vi "measure_test.vi"() -> ()   [LabVIEW 2019]
panel:
  in  "dir & target 13":T1 {"Target (cm||deg)" format="%#_13g"}
  in  "dir & target 12":T1 {"Target (cm||deg)" format="%#_13g"}
  in  "dir & target 11":T1 {"Target (cm||deg)" format="%#_13g"}
  in  "dir & target 10":T1 {"Target (cm||deg)" format="%#_13g"}
  in  "dir & target 9":T1 {"Target (cm||deg)" format="%#_13g"}
  in  "dir & target 8":T1 {"Target (cm||deg)" format="%#_13g"}
  in  "dir & target 7":T1={"direction"=enum."Tilt(R)", "Target (cm||deg)"=-73.0} {"Target (cm||deg)" format="%#_13g"}
  in  "dir & target 6":T1={"direction"=enum."Tilt(R)", "Target (cm||deg)"=-73.0} {"Target (cm||deg)" format="%#_13g"}
  in  "dir & target 5":T1={"direction"=enum."Forward", "Target (cm||deg)"=-69.2} {"Target (cm||deg)" format="%#_13g"}
  in  "dir & target 4":T1={"direction"=enum."Tilt(R)", "Target (cm||deg)"=-73.0} {"Target (cm||deg)" format="%#_13g"}
  in  "dir & target 3":T1={"direction"=enum."Forward", "Target (cm||deg)"=-69.2} {"Target (cm||deg)" format="%#_13g"}
  in  "dir & target 2":T1={"direction"=enum."Tilt(R)", "Target (cm||deg)"=122.0} {"Target (cm||deg)" format="%#_13g"}
  in  "dir & target 1":T1={"direction"=enum."Tilt(R)", "Target (cm||deg)"=-128.0} {"Target (cm||deg)" format="%#_13g"}
  in  "dir & target":T1={"direction"=enum."Forward", "Target (cm||deg)"=307.0} {"Target (cm||deg)" format="%#_13g"}
  out "error out":errorcluster
  in  "error in (no error)":errorcluster
  # "Out bridge"
  # "In bridge"
  # "In bridge"
  # "Out bridge"
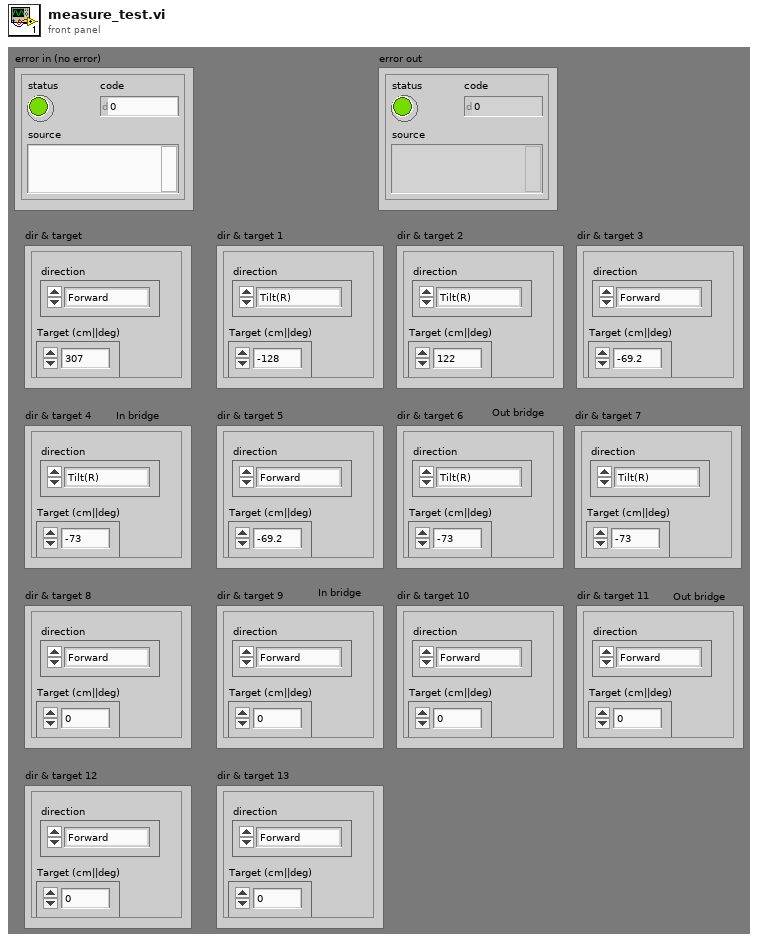
[diagram p1: front panel]
types:
  T1 = cluster{"direction":enum16{"Forward", "Tilt(R)", "Turn"}, "Target (cm||deg)":dbl}
  T2 = enum16{"LeftDown", "LeftUp", "RightDown", "RightUp", "Right", "Left", "Up", "Down", "Middle(X)", "Middle(Y)"}
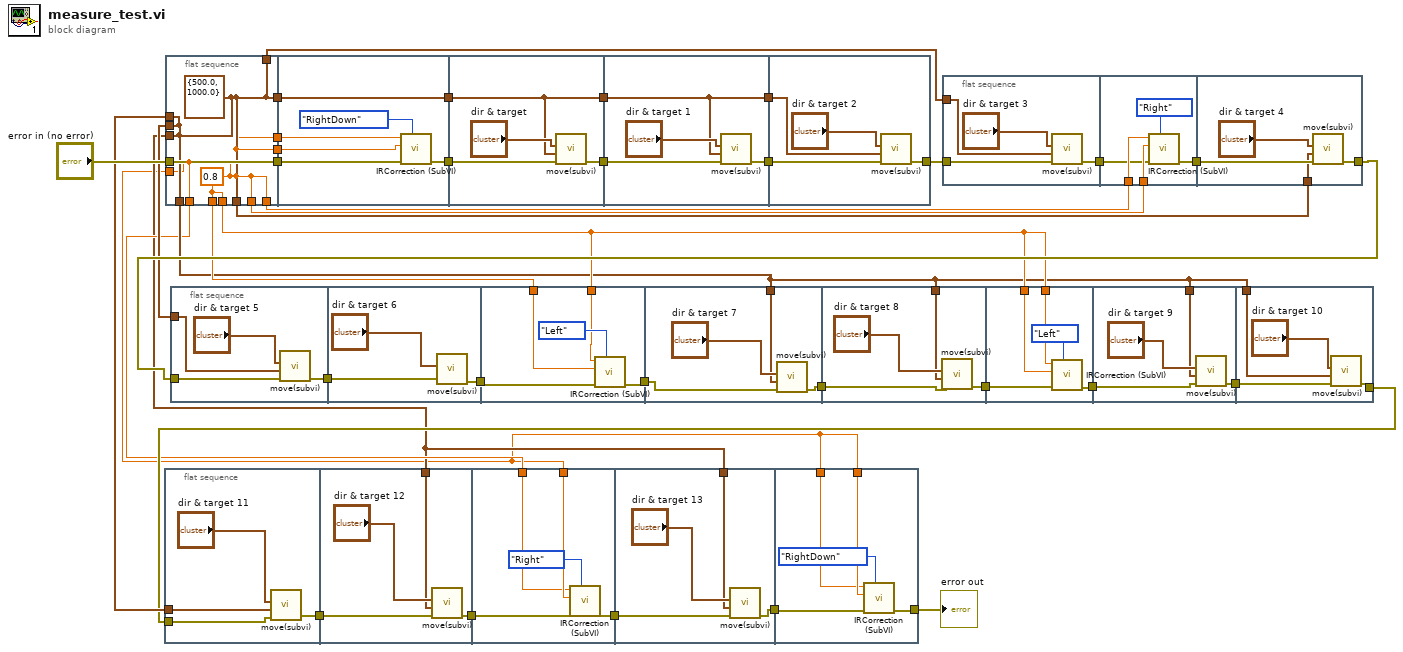
[diagram p0: block diagram]
diagram:
  n1 = flat-sequence {
    tunnel: w10 -> [w43]
    tunnel: w9 -> [w42]
    tunnel: [w41] -> w8
    tunnel: w8 -> [w48]
    tunnel: w3 -> [w46]
    tunnel: [w45] -> w7
    tunnel: w7 -> [w53]
    tunnel: w1 -> [w52]
    tunnel: w6 -> [w51]
    tunnel: [w49] -> w5
    tunnel: w5 -> [w57]
    tunnel: w3 -> [w54]
    tunnel: [w56] -> w2
    tunnel: [w61] -> w4
    tunnel: w2 -> [w62]
    tunnel: w1 -> [w60]
    tunnel: w1 -> [w59]
    frame #0 {
      n2 = call "move(subvi).vi"("Error In"=w42, "speed"=w43, "dir & target"="dir & target 11") -> ("Error Out"=w41:errorcluster)  [unwired: 8 in]
    }
    frame #1 {
      n3 = call "move(subvi).vi"("Error In"=w48, "speed"=w46, "dir & target"="dir & target 12") -> ("Error Out"=w45:errorcluster)  [unwired: 8 in]
    }
    frame #2 {
      n4 = call "IRCorrection (SubVI).vi"("CorrectCorner"=T2."Right", "error in (no error)"=w53, "Y_distance(V)"=w52, "X_distance(V)"=w51) -> ("error out"=w49:errorcluster)  [unwired: 6 in, 1 out]
    }
    frame #3 {
      n5 = call "move(subvi).vi"("Error In"=w57, "speed"=w54, "dir & target"="dir & target 13") -> ("Error Out"=w56:errorcluster)  [unwired: 8 in]
    }
    frame #4 {
      n6 = call "IRCorrection (SubVI).vi"("CorrectCorner"=T2."RightDown", "error in (no error)"=w62, "Y_distance(V)"=w60, "X_distance(V)"=w59) -> ("error out"=w61:errorcluster)  [unwired: 6 in, 1 out]
    }
  }
  n7 = flat-sequence {
    tunnel: [w63] -> w40
    tunnel: [w63] -> w39
    tunnel: "error in (no error)" -> [w65]
    tunnel: [w65] -> w38
    tunnel: [w64] -> w35
    tunnel: [w64] -> w29
    tunnel: [w63] -> w27
    tunnel: [w63] -> w26
    tunnel: [w64] -> w23
    tunnel: [w64] -> w20
    tunnel: [w63] -> w17
    tunnel: [w63] -> w14
    tunnel: [w64] -> w11
    tunnel: [w64] -> w10
    tunnel: [w64] -> w3
    tunnel: [w63] -> w1
    tunnel: [w63] -> w6
    tunnel: w40 -> [w70]
    tunnel: w39 -> [w69]
    tunnel: w38 -> [w68]
    tunnel: [w67] -> w36
    tunnel: w35 -> [w67]
    tunnel: [w66] -> w34
    tunnel: w36 -> [w72]
    tunnel: w34 -> [w74]
    tunnel: [w73] -> w33
    tunnel: [w72] -> w32
    tunnel: w33 -> [w79]
    tunnel: w32 -> [w76]
    tunnel: [w77] -> w31
    tunnel: [w76] -> w30
    tunnel: w31 -> [w83]
    tunnel: w30 -> [w82]
    tunnel: [w80] -> w28
    frame #0 {
      w64 = cluster{"acc (deg/s^2)":dbl, "Vmax (deg/s)":dbl} {"acc (deg/s^2)"=500.0, "Vmax (deg/s)"=1000.0} ("speed")
      w63 = 0.8 ("X_distance(V)")
    }
    frame #1 {
      n8 = call "IRCorrection (SubVI).vi"("CorrectCorner"=T2."RightDown", "error in (no error)"=w68, "Y_distance(V)"=w69, "X_distance(V)"=w70) -> ("error out"=w66:errorcluster)  [unwired: 6 in, 1 out]
    }
    frame #2 {
      n9 = call "move(subvi).vi"("Error In"=w74, "speed"=w72, "dir & target"="dir & target") -> ("Error Out"=w73:errorcluster)  [unwired: 8 in]
    }
    frame #3 {
      n10 = call "move(subvi).vi"("Error In"=w79, "speed"=w76, "dir & target"="dir & target 1") -> ("Error Out"=w77:errorcluster)  [unwired: 8 in]
    }
    frame #4 {
      n11 = call "move(subvi).vi"("Error In"=w83, "speed"=w82, "dir & target"="dir & target 2") -> ("Error Out"=w80:errorcluster)  [unwired: 8 in]
    }
  }
  n12 = flat-sequence {
    tunnel: w20 -> [w86]
    tunnel: w21 -> [w85]
    tunnel: [w84] -> w22
    tunnel: w22 -> [w89]
    tunnel: [w88] -> w19
    tunnel: w19 -> [w95]
    tunnel: [w94] -> w18
    tunnel: w17 -> [w92]
    tunnel: w14 -> [w91]
    tunnel: w18 -> [w98]
    tunnel: w11 -> [w97]
    tunnel: [w96] -> w16
    tunnel: w16 -> [w103]
    tunnel: w11 -> [w101]
    tunnel: [w100] -> w15
    tunnel: w15 -> [w108]
    tunnel: w14 -> [w107]
    tunnel: w14 -> [w106]
    tunnel: [w105] -> w13
    tunnel: w13 -> [w112]
    tunnel: [w111] -> w12
    tunnel: w11 -> [w109]
    tunnel: w12 -> [w116]
    tunnel: w11 -> [w114]
    tunnel: [w113] -> w9
    frame #0 {
      n13 = call "move(subvi).vi"("Error In"=w85, "speed"=w86, "dir & target"="dir & target 5") -> ("Error Out"=w84:errorcluster)  [unwired: 8 in]
    }
    frame #1 {
      n14 = call "move(subvi).vi"("Error In"=w89, "dir & target"="dir & target 6") -> ("Error Out"=w88:errorcluster)  [unwired: 9 in]
    }
    frame #2 {
      n15 = call "IRCorrection (SubVI).vi"("CorrectCorner"=T2."Left", "error in (no error)"=w95, "Y_distance(V)"=w92, "X_distance(V)"=w91) -> ("error out"=w94:errorcluster)  [unwired: 6 in, 1 out]
    }
    frame #3 {
      n16 = call "move(subvi).vi"("Error In"=w98, "speed"=w97, "dir & target"="dir & target 7") -> ("Error Out"=w96:errorcluster)  [unwired: 8 in]
    }
    frame #4 {
      n17 = call "move(subvi).vi"("Error In"=w103, "speed"=w101, "dir & target"="dir & target 8") -> ("Error Out"=w100:errorcluster)  [unwired: 8 in]
    }
    frame #5 {
      n18 = call "IRCorrection (SubVI).vi"("CorrectCorner"=T2."Left", "error in (no error)"=w108, "Y_distance(V)"=w106, "X_distance(V)"=w107) -> ("error out"=w105:errorcluster)  [unwired: 6 in, 1 out]
    }
    frame #6 {
      n19 = call "move(subvi).vi"("Error In"=w112, "speed"=w109, "dir & target"="dir & target 9") -> ("Error Out"=w111:errorcluster)  [unwired: 8 in]
    }
    frame #7 {
      n20 = call "move(subvi).vi"("Error In"=w116, "speed"=w114, "dir & target"="dir & target 10") -> ("Error Out"=w113:errorcluster)  [unwired: 8 in]
    }
  }
  n21 = flat-sequence {
    tunnel: w29 -> [w119]
    tunnel: w28 -> [w118]
    tunnel: [w117] -> w25
    tunnel: w27 -> [w125]
    tunnel: w26 -> [w124]
    tunnel: w25 -> [w123]
    tunnel: [w122] -> w24
    tunnel: w24 -> [w129]
    tunnel: [w128] -> w21
    tunnel: w23 -> [w126]
    frame #0 {
      n22 = call "move(subvi).vi"("Error In"=w118, "speed"=w119, "dir & target"="dir & target 3") -> ("Error Out"=w117:errorcluster)  [unwired: 8 in]
    }
    frame #1 {
      n23 = call "IRCorrection (SubVI).vi"("CorrectCorner"=T2."Right", "error in (no error)"=w123, "Y_distance(V)"=w124, "X_distance(V)"=w125) -> ("error out"=w122:errorcluster)  [unwired: 6 in, 1 out]
    }
    frame #2 {
      n24 = call "move(subvi).vi"("Error In"=w129, "speed"=w126, "dir & target"="dir & target 4") -> ("Error Out"=w128:errorcluster)  [unwired: 8 in]
    }
  }
  "error out" <- w4
